vi "DWF PS Configure Current Output.vi"(0 "Instrument Handle In":u32, 5 "Channel":string, 7 "Current Level":dbl=0.1 caption="Current Level (no change)", 9 "Voltage Limit":dbl caption="Voltage Limit (no change)", 11 "Error In":errorcluster caption="Error In (no error)") -> (4 "Instrument Handle Out":u32, 15 "Error Out":errorcluster)   [LabVIEW 2015, in "DigilentWF.lvlib"]
doc: "Configures a current output on the specified channel. This VI should be called once for every channel you want to configure to output current."
uses:
  <vilib>/DigilentWF/DigilentWF.lvlib
  dwf.dll
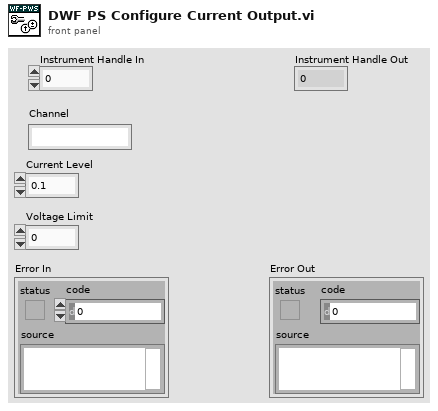
[diagram p1: front panel]
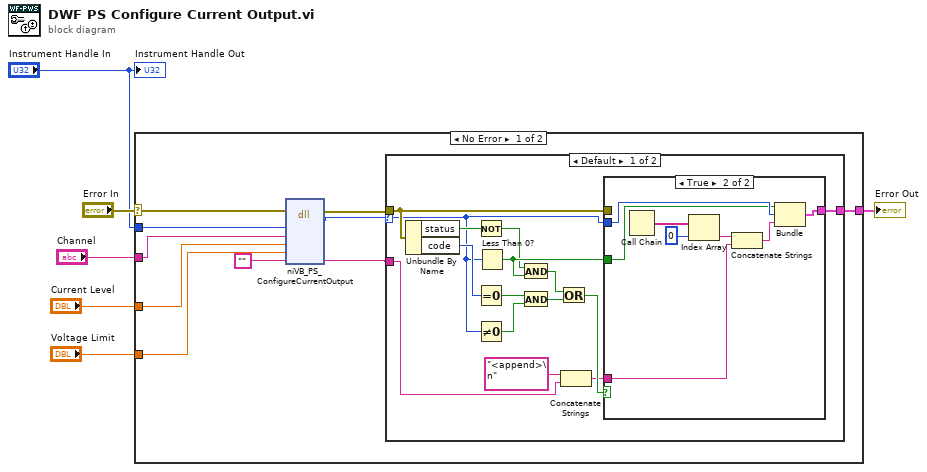
[diagram p0: block diagram]
diagram:
  n1 = case "outter_case" shown="No Error" "Error In" {
    selector: "Error In" -> [w15 w42]
    tunnel: [w16 w42] -> w5
    tunnel: "Instrument Handle In" -> [w14 _]
    tunnel: "Current Level" -> [w13 _]
    tunnel: "Voltage Limit" -> [w12 _]
    tunnel: "Channel" -> [w7 _]
    frame No Error {
      n2 = dll-call lib="dwf.*" fn="niVB_PS_ConfigureCurrentOutput"(error in=w15, "instrumentHandle"=w14, "channel"=w7, "currentLevel"=w13, "voltageLimit"=w12, "szError"="") -> (error out=w11:errorcluster, "return type"=w10:u32, "szError"=w9:string)  [unwired: 6 in, 1 out]
      n3 = case "inner_case" shown="Default" w10 {
        selector: w10 -> [w21 _]
        tunnel: w11 -> [w22 w41]
        tunnel: [w18 w41] -> w16
        tunnel: w9 -> [w17 _]
        frame Default {
          n4 = Unbundle By Name(w22) -> ("status"=w26:bool, "code"=w30:i32)
          n5 = Not(x=w26) -> (.not. x?=w29:bool)
          n6 = Equal To 0?(x=w30) -> (x = 0?=w25:bool)
          n7 = Not Equal To 0?(x=w21) -> (x != 0?=w28:bool)
          n8 = Less Than 0?(x=w21) -> (x < 0?=w31:bool)
          n9 = And(x=w29, y=w31) -> (x .and. y?=w27:bool)
          n10 = And(x=w25, y=w28) -> (x .and. y?=w24:bool)
          n11 = Or(x=w27, y=w24) -> (x .or. y?=w23:bool)
          n12 = Concatenate Strings("<append>\n" ("string"), w17) -> (w20:string)
          n13 = case shown="True" w23 {
            tunnel: [w32 w39] -> w18
            tunnel: w21 -> [_ w38]
            tunnel: w31 -> [_ w37]
            tunnel: w22 -> [w32 _]
            tunnel: w20 -> [_ w33]
            frame False {
            }
            frame True {
              n14 = Call Chain() -> (call chain=w36:string[])
              n15 = Index Array(array=w36, index=0) -> (element=w35:string)
              n16 = Concatenate Strings(w35, w33) -> (w40:string)
              n17 = Bundle(w37, "return type"=w38, w40) -> (w39:cluster{bool, "return type":u32, string})  [unwired: 1 out]
            }
          }
        }
        frame 0 {
        }
      }
    }
    frame Error {
    }
  }
  "Error Out" <- w5
  "Instrument Handle Out" <- "Instrument Handle In"
